vi "Config.vi"() -> ()   [LabVIEW 2020]
uses:
  Global_Variable/Global.vi
  Global_Variable/A180648.vi
  <vilib>/Utility/config.llb/NI_LVConfig.lvlib
  Libraries/S7/S7.lvlib
panel:
  in  "实验项":T1
  in  "滑移力复测":bool
  in  "产品型号":string(combo)
  in  "删除":bool
  in  "确定":bool
  in  "添加":bool
  in  "退出":bool
  in  "更新":bool
  in  "选项卡控件":enum32{"产品参数"}(tab)
  in  "结果判定参数":string[][](table)=[["mm"], ["KN"], ["KN"], ["KN"], [""], [""], [""], [""], [""], [""], [""], [""]]
  in  "判定框参数":string[][](table)=[["mm"], ["KN"], ["mm"], ["KN"]]
  in  "坐标轴参数":string[][](table)=[[""], ["°/S"], ["°"], ["Nm"]]
  # "滑移力复测及管柱总成装配台"
types:
  T1 = cluster{"第一颗螺丝":bool, "第二颗螺丝":bool, "第三颗螺丝 ":bool}
  T2 = typedef "NI_LVConfig.lvlib/Config Data RefNum.ctl" = refnum<k1>
  T3 = cluster{"[0]":cluster{string, dbl, dbl}, "[1]":cluster{string, dbl, dbl}, "[2]":cluster{string, dbl, dbl}, "[3]":cluster{string, dbl, dbl}}
  T4 = cluster{"位移":cluster{"单位":string, "下限":dbl, "上限":dbl}, "拉力":cluster{"单位":string, "下限":dbl, "上限":dbl}, "位移1":cluster{"单位":string, "下限":dbl, "上限":dbl}, "压力":cluster{"单位":string, "下限":dbl, "上限":dbl}}
  T5 = cluster{"[0]":cluster{string, dbl, dbl}, "[1]":cluster{string, dbl, dbl}, "[2]":cluster{string, dbl, dbl}, "[3]":cluster{string, dbl, dbl}, "[4]":cluster{string, dbl, dbl}, "[5]":cluster{string, dbl, dbl}}
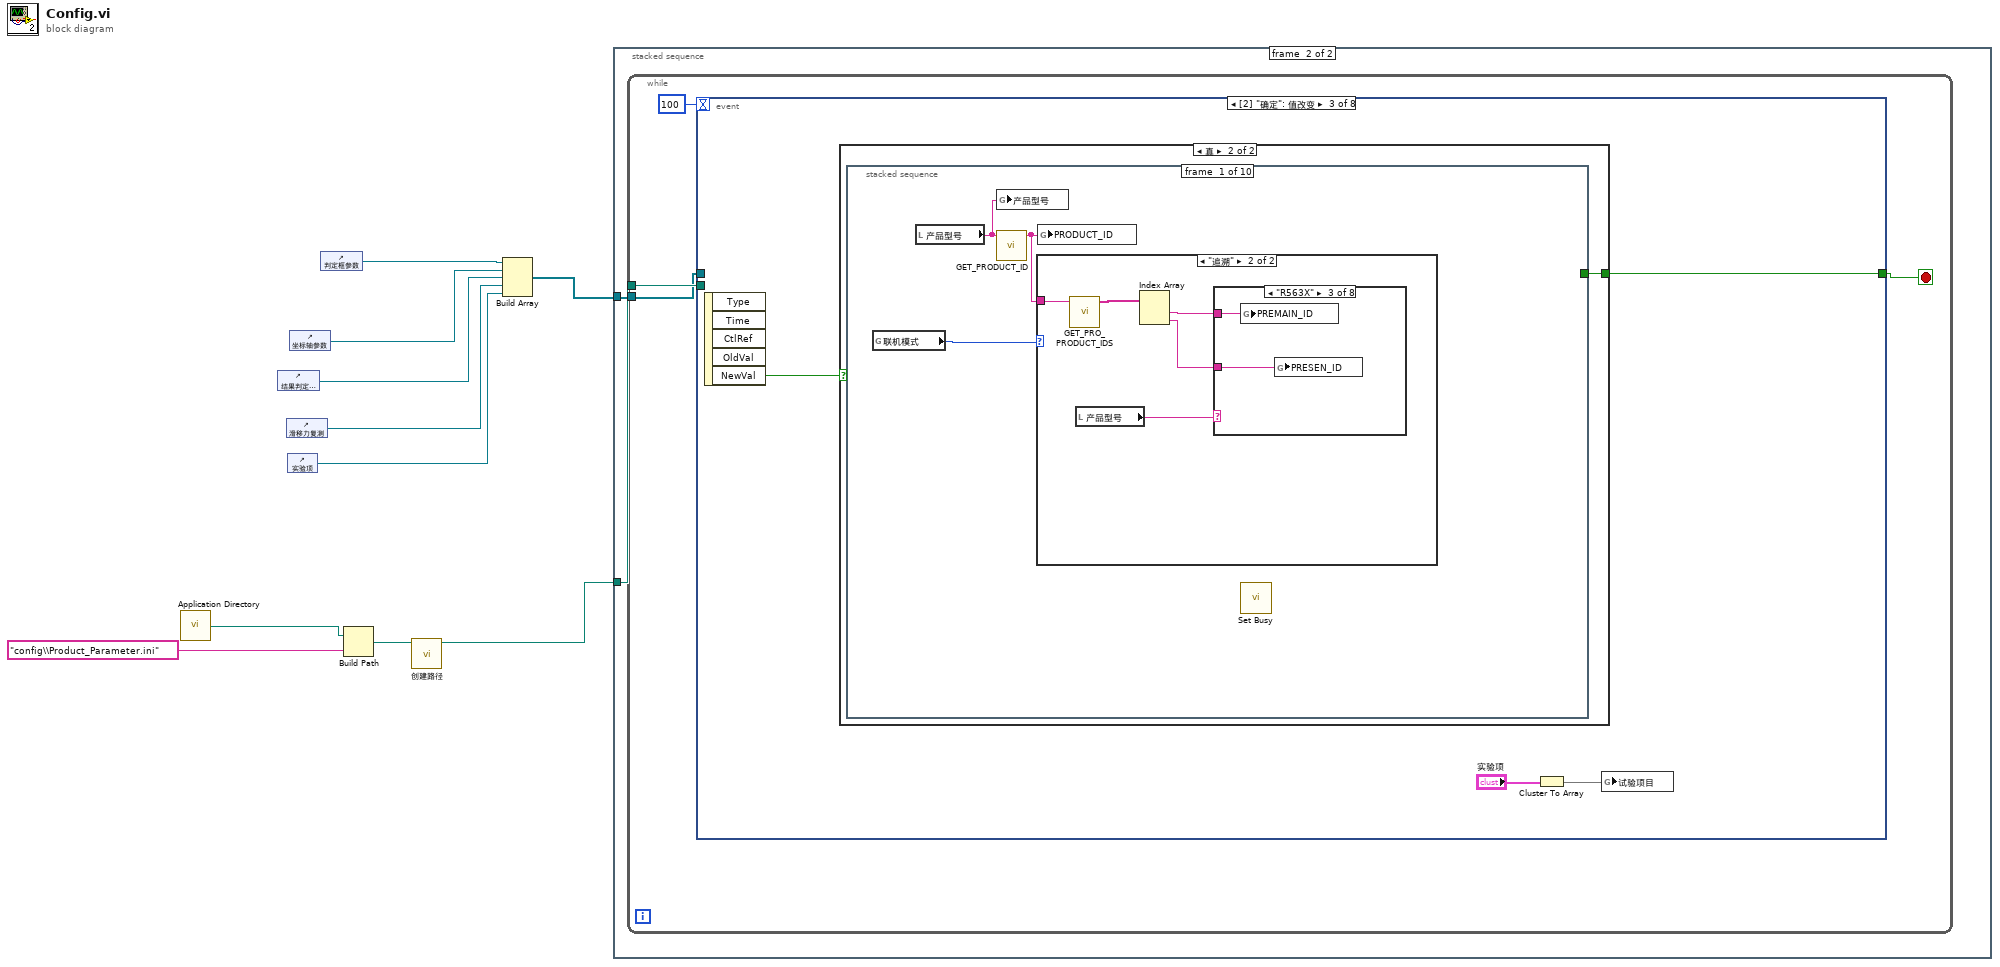
[diagram p0: block diagram]
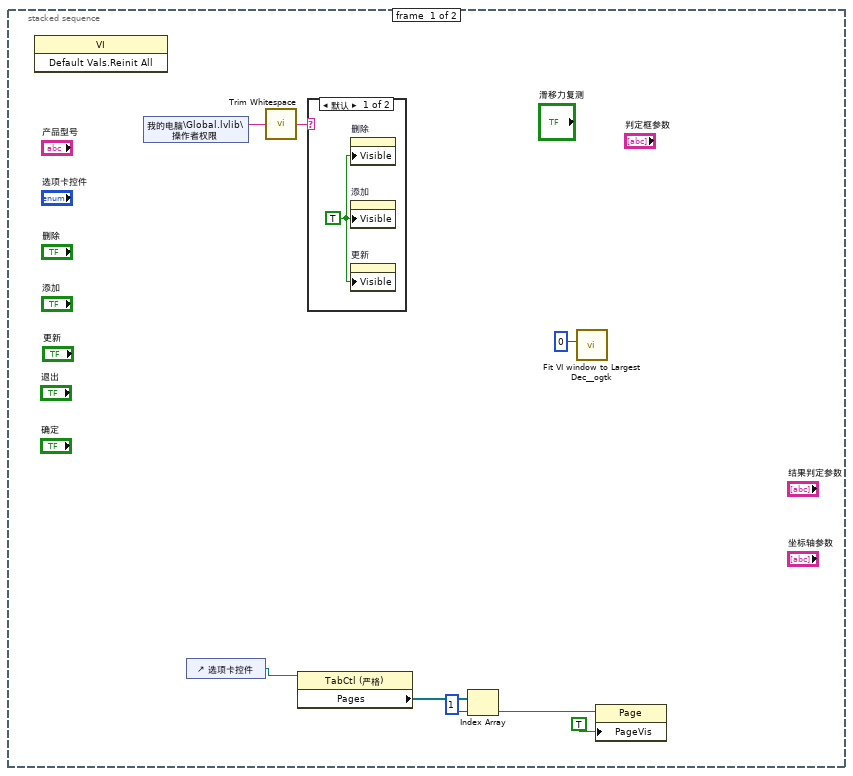
[diagram p2: hidden frame]
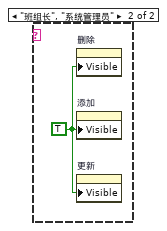
[diagram p3: hidden frame]
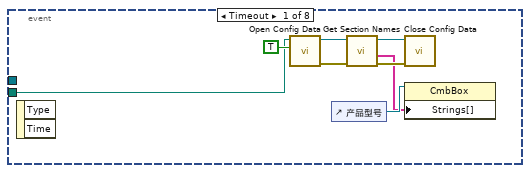
[diagram p4: hidden frame]
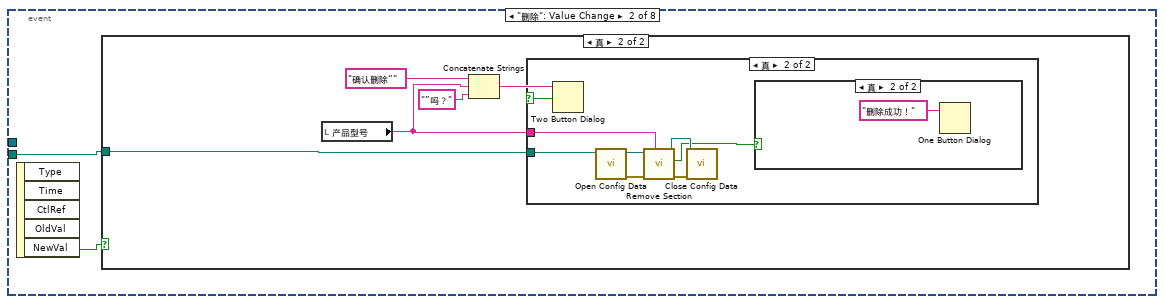
[diagram p5: hidden frame]
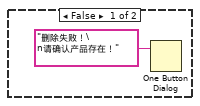
[diagram p8: hidden frame]
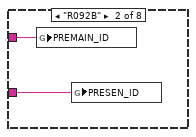
[diagram p12: hidden frame]
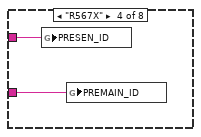
[diagram p13: hidden frame]
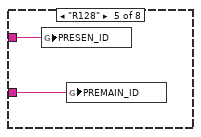
[diagram p14: hidden frame]
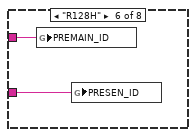
[diagram p15: hidden frame]
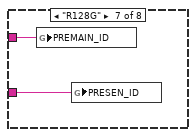
[diagram p16: hidden frame]
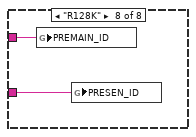
[diagram p17: hidden frame]
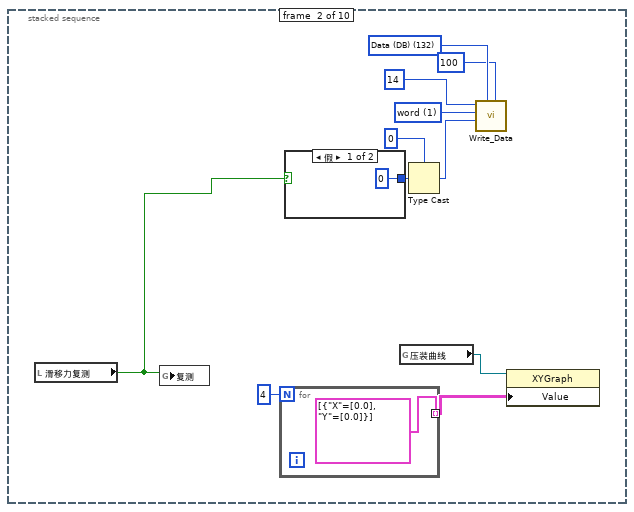
[diagram p18: hidden frame]
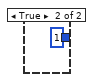
[diagram p19: hidden frame]
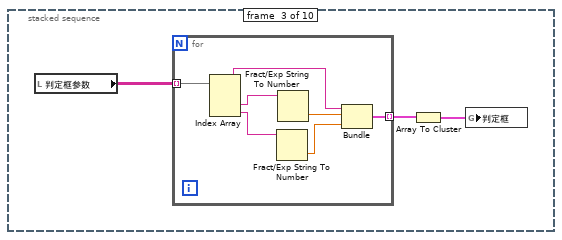
[diagram p20: hidden frame]
diagram:
  n1 = call <vilib>:"Application Directory.vi"() -> ("Application Directory"=w9:path)
  n2 = control-ref of="结果判定参数"() -> (w4:refnum<vi>)
  n3 = control-ref of="滑移力复测"() -> (w2:refnum<vi>)
  n4 = control-ref of="实验项"() -> (w1:refnum<vi>)
  n5 = control-ref of="坐标轴参数"() -> (w5:refnum<vi>)
  n6 = control-ref of="判定框参数"() -> (w3:refnum<vi>)
  n7 = Build Path(base path=w9, name or relative path="config\\Product_Parameter.ini" ("名称或相对路径")) -> (appended path=w7:path)
  n8 = call "创建路径.vi"("path"=w7) -> ("path out"=w6:path)  [unwired: 9 in, 1 out]
  n9 = Build Array(w3, w5, w4, w2, w1) -> (w10:refnum<vi>[])
  n10 = stacked-sequence {
    tunnel: w10 -> [_ w22]
    tunnel: w6 -> [_ w21]
    frame #0 {
      n11 = invoke class="VI" method="Default Vals.Reinit All"() -> ()  [unwired: 3 in, 3 out]
      n12 = shared-variable "我的电脑\\Global.lvlib\\操作者权限"() -> (w18:string)  [unwired: 1 in, 1 out]
      n13 = control-ref of="选项卡控件"() -> (w15:refnum<vi>)
      n14 = call <vilib>:"Trim Whitespace.vi"("string"=w18) -> ("trimmed string"=w17:string)  [unwired: 1 in]
      n15 = property class="TabCtl (严格)"(reference=w15) -> ("Pages"=w14:refnum<vi>[])  [unwired: 1 in, 2 out]
      n16 = case shown="默认" w17 {
        frame Default {
          w19 = TRUE ("可见")
          n17 = property on="删除" class="Bool (严格)"("Visible"=w19) -> ()  [unwired: 2 in, 2 out]
          n18 = property on="添加" class="Bool (严格)"("Visible"=w19) -> ()  [unwired: 2 in, 2 out]
          n19 = property on="更新" class="Bool (严格)"("Visible"=w19) -> ()  [unwired: 2 in, 2 out]
        }
        frame "班组长", "系统管理员" {
          w20 = TRUE ("可见")
          n20 = property on="删除" class="Bool (严格)"("Visible"=w20) -> ()  [unwired: 2 in, 2 out]
          n21 = property on="添加" class="Bool (严格)"("Visible"=w20) -> ()  [unwired: 2 in, 2 out]
          n22 = property on="更新" class="Bool (严格)"("Visible"=w20) -> ()  [unwired: 2 in, 2 out]
        }
      }
      n23 = Index Array(array=w14, index=1 ("索引")) -> (element=w13:refnum<vi>)
      n24 = call <userlib>:"Fit VI window to Largest Dec__ogtk.vi"("border spacing (2 px)"=0) -> ()  [unwired: 5 in, 2 out]
      n25 = property class="Page"(reference=w13, "PageVis"=TRUE ("选项卡可见")) -> ()  [unwired: 1 in, 2 out]
    }
    frame #1 {
      n26 = while {
        tunnel: w21 -> [w26]
        tunnel: w22 -> [w24]
        stop <- w25 stop-if-true
        n27 = event shown="[2] \"确定\": 值改变" {
          selector: _ -> [_ _ _ _ _ _ _ _]
          dyn-events: _ -> [_ _ _ _ _ _ _ _]
          timeout: 100 -> [_ _ _ _ _ _ _ _]
          tunnel: w26 -> [w29 w36 _ w158 w185 _ w209 _]
          tunnel: [_ _ w54 _ _ TRUE _ TRUE] -> w25
          tunnel: w24 -> [_ _ _ w159 w186 _ w208 _]
          event Timeout {
            n28 = event-data() -> ()  [unwired: 1 in, 2 out]
            n29 = call <vilib>:"Open Config Data.vi"("create file if necessary (T)"=TRUE, "configuration file path"=w29) -> ("error out"=w31:errorcluster, "refnum"=w30:T2)  [unwired: 7 in, 1 out]
            n30 = control-ref of="产品型号"() -> (w28:refnum<vi>)
            n31 = call <vilib>:"Get Section Names.vi"("error in (no error)"=w31, "refnum"=w30) -> ("error out"=w33:errorcluster, "section names"=w27:string[], "refnum out"=w32:T2)  [unwired: 7 in]
            n32 = call <vilib>:"Close Config Data.vi"("error in (no error)"=w33, "refnum"=w32) -> ()  [unwired: 8 in, 2 out]
            n33 = property on="属性节点" class="CmbBox"(reference=w28, "Strings[]"=w27) -> ()  [unwired: 1 in, 2 out]
          }
          event "删除": Value Change {
            n34 = event-data() -> ("NewVal"=w35:bool)  [unwired: 1 in, 4 out]
            n35 = case shown="真" w35 {
              tunnel: w36 -> [_ w38]
              frame False {
              }
              frame True {
                n36 = local read "产品型号"() -> (w37:string)
                n37 = Concatenate Strings("确认删除“", w37, "”吗？") -> (w40:string)
                n38 = Two Button Dialog(message=w40) -> (T button?=w39:bool)  [unwired: 2 in]
                n39 = case shown="真" w39 {
                  tunnel: w38 -> [_ w44]
                  tunnel: w37 -> [_ w43]
                  frame False {
                  }
                  frame True {
                    n40 = call <vilib>:"Open Config Data.vi"("configuration file path"=w44) -> ("error out"=w46:errorcluster, "refnum"=w49:T2)  [unwired: 8 in, 1 out]
                    n41 = call <vilib>:"Remove Section.vi"("section"=w43, "error in (no error)"=w46, "refnum"=w49) -> ("error out"=w48:errorcluster, "section exists?"=w45:bool, "refnum out"=w47:T2)  [unwired: 6 in]
                    n42 = call <vilib>:"Close Config Data.vi"("error in (no error)"=w48, "refnum"=w47) -> ()  [unwired: 8 in, 2 out]
                    n43 = case shown="真" w45 {
                      frame False {
                        n44 = One Button Dialog(message="删除失败！\n请确认产品存在！" ("消息")) -> ()  [unwired: 1 in, 1 out]
                      }
                      frame True {
                        n45 = One Button Dialog(message="删除成功！" ("消息")) -> ()  [unwired: 1 in, 1 out]
                      }
                    }
                  }
                }
              }
            }
          }
          event "确定": Value Change {
            n46 = event-data() -> ("NewVal"=w55:bool)  [unwired: 1 in, 4 out]
            n47 = case shown="真" w55 {
              tunnel: [_ w56] -> w54
              frame False {
              }
              frame True {
                n48 = stacked-sequence {
                  tunnel: [_ _ _ _ _ _ _ _ _ TRUE] -> w56
                  frame #0 {
                    n49 = global read "Global.vi" "联机模式"() -> (w57:enum16{"单机", "追溯"})
                    n50 = local read "产品型号"() -> (w59:string)
                    n51 = global write "Global.vi" "产品型号"(w59) -> ()
                    n52 = call "GET_PRODUCT_ID.vi"("PRODFUCT_NAME"=w59) -> ("PRODUCT_ID"=w58:string)  [unwired: 10 in]
                    n53 = case shown="\"追溯\"" w57 {
                      tunnel: w58 -> [_ w64]
                      frame "单机", Default {
                      }
                      frame "追溯" {
                        n54 = call "GET_PRO_PRODUCT_IDS.vi"("PRODUCT_ID"=w64) -> ("前序工位"=w63:string[])  [unwired: 10 in]
                        n55 = local read "产品型号"() -> (w60:string)
                        n56 = Index Array(array=w63) -> (element #1=w62:string, element #2=w61:string)  [unwired: 2 in]
                        n57 = case shown="\"R563X\"" w60 {
                          tunnel: w62 -> [_ w66 w68 w70 w72 w74 w76 w78]
                          tunnel: w61 -> [_ w65 w67 w69 w71 w73 w75 w77]
                          frame "假", Default {
                          }
                          frame "R092B" {
                            n58 = global write "追溯Global.vi" "PREMAIN_ID"(w66) -> ()
                            n59 = global write "追溯Global.vi" "PRESEN_ID"(w65) -> ()
                          }
                          frame "R563X" {
                            n60 = global write "追溯Global.vi" "PREMAIN_ID"(w68) -> ()
                            n61 = global write "追溯Global.vi" "PRESEN_ID"(w67) -> ()
                          }
                          frame "R567X" {
                            n62 = global write "追溯Global.vi" "PRESEN_ID"(w70) -> ()
                            n63 = global write "追溯Global.vi" "PREMAIN_ID"(w69) -> ()
                          }
                          frame "R128" {
                            n64 = global write "追溯Global.vi" "PRESEN_ID"(w72) -> ()
                            n65 = global write "追溯Global.vi" "PREMAIN_ID"(w71) -> ()
                          }
                          frame "R128H" {
                            n66 = global write "追溯Global.vi" "PREMAIN_ID"(w74) -> ()
                            n67 = global write "追溯Global.vi" "PRESEN_ID"(w73) -> ()
                          }
                          frame "R128G" {
                            n68 = global write "追溯Global.vi" "PREMAIN_ID"(w76) -> ()
                            n69 = global write "追溯Global.vi" "PRESEN_ID"(w75) -> ()
                          }
                          frame "R128K" {
                            n70 = global write "追溯Global.vi" "PREMAIN_ID"(w78) -> ()
                            n71 = global write "追溯Global.vi" "PRESEN_ID"(w77) -> ()
                          }
                        }
                      }
                    }
                    n72 = global write "追溯Global.vi" "PRODUCT_ID"(w58) -> ()
                    n73 = call <vilib>:"Set Busy.vi"() -> ()  [unwired: 10 in, 2 out]
                  }
                  frame #1 {
                    w84 = u16 1 items=["byte", "word", "Dword"] ("数据类型")
                    w86 = u8 132 items=["I/O (P)"=128, "Input (I)"=129, "Output (Q)"=130, "Bit Memory (M)"=131, "Data (DB)"=132, "Instance Data (DI)"=133, "Local Data (L)"=134, "Predecessor Local Data (VL)"=135] ("寄存器类型")
                    n74 = local read "滑移力复测"() -> (w79:bool)
                    n75 = global write "Global.vi" "复测"(w79) -> ()
                    n76 = for {
                      N: 4 -> [_]
                      tunnel: [cluster{"X":dbl[], "Y":dbl[]}[] [{"X"=[0.0], "Y"=[0.0]}]] -> w89 mode=indexing
                    }
                    n77 = case shown="假" w79 {
                      tunnel: [0 ("x") 1 ("x")] -> w80
                      frame False {
                      }
                      frame True {
                      }
                    }
                    n78 = global read "A180648.vi" "压装曲线"() -> (w87:refnum<vi>)
                    n79 = Type Cast(type=u32 0 ("写入地址"), x=w80) -> (*(type *) &x=w82:u32)
                    n80 = call "Write_Data.vi"("DB #"=u16 100, "寄存器类型"=w86, "写入数据"=w82, "数据类型"=w84, "写入地址"=u32 14) -> ()  [unwired: 4 in, 3 out]
                    n81 = property class="XYGraph"(reference=w87, "Value"=w89) -> ()  [unwired: 1 in, 2 out]
                  }
                  frame #2 {
                    n82 = local read "判定框参数"() -> (w95:string[][])
                    n83 = for {
                      tunnel: w95 -> [w102] mode=indexing
                      tunnel: [w96] -> w94 mode=indexing
                      n84 = Index Array(array=w102) -> (element #1=w99:string, element #2=w101:string, element #3=w100:string)  [unwired: 3 in]
                      n85 = Fract/Exp String To Number(string=w100) -> (number=w97:dbl)  [unwired: 3 in, 1 out]
                      n86 = Fract/Exp String To Number(string=w101) -> (number=w98:dbl)  [unwired: 3 in, 1 out]
                      n87 = Bundle(w99, w98, w97) -> (w96:cluster{string, dbl, dbl})  [unwired: 1 in]
                    }
                    n88 = Array To Cluster(array=w94) -> (cluster=w93:T3)
                    n89 = global write "判定参数.vi" "判定框"(w93) -> ()
                  }
                  frame #3 {
                    n90 = global read "A180648.vi" "压装曲线"() -> (w109:refnum<vi>)
                    n91 = property class="XYGraph"(reference=w109) -> (reference out=w106:refnum<vi>, "Value"=w108:variant)  [unwired: 1 in, 1 out]
                    n92 = Variant To Data(type=cluster{"X":dbl[], "Y":dbl[]}[] [{"X"=[], "Y"=[]}], Variant=w108) -> (data=w107:cluster{"X":dbl[], "Y":dbl[]}[])  [unwired: 1 in, 1 out]
                    n93 = global read "判定参数.vi" "判定框"() -> (w103:T4)
                    n94 = for {
                      tunnel: w107 -> [w112] mode=indexing
                      tunnel: [w111] -> w104 mode=indexing
                      tunnel: w103 -> [w110]
                      i -> [w113]
                      n95 = case shown="1" w113 {
                        tunnel: w112 -> [w114 _ _]
                        tunnel: [w114 w117 w127] -> w111
                        tunnel: w110 -> [_ w122 w128]
                        frame Default {
                        }
                        frame 0 {
                          n96 = Unbundle By Name(w122) -> ("位移.下限"=w121:dbl, "位移.上限"=w120:dbl, "压力.下限"=w115:dbl, "压力.上限"=w116:dbl)
                          n97 = Build Array(w120, w120, w121, w121, w120) -> (w119:dbl[])
                          n98 = Build Array(w115, w116, w116, w115, w115) -> (w118:dbl[])
                          n99 = Bundle(w119, w118) -> (w117:cluster{dbl[], dbl[]})  [unwired: 1 in]
                        }
                        frame 1 {
                          n100 = Unbundle By Name(w128) -> ("位移.下限"=w132:dbl, "位移.上限"=w131:dbl, "压力.上限"=w125:dbl, "压力.下限"=w126:dbl)
                          n101 = Negate(x=w126) -> (-x=w123:dbl)
                          n102 = Negate(x=w125) -> (-x=w124:dbl)
                          n103 = Build Array(w131, w131, w132, w132, w131) -> (w130:dbl[])
                          n104 = Build Array(w124, w123, w123, w124, w124) -> (w129:dbl[])
                          n105 = Bundle(w130, w129) -> (w127:cluster{dbl[], dbl[]})  [unwired: 1 in]
                        }
                      }
                    }
                    n106 = property class="XYGraph"(reference=w106, "Value"=w104) -> ()  [unwired: 1 in, 2 out]
                  }
                  frame #4 {
                    n107 = local read "结果判定参数"() -> (w135:string[][])
                    n108 = for {
                      tunnel: w135 -> [w137] mode=indexing
                      tunnel: [w136] -> w133 mode=indexing
                      n109 = Index Array(array=w137) -> (element #1=w142:string, element #2=w141:string, element #3=w139:string)  [unwired: 3 in]
                      n110 = Fract/Exp String To Number(string=w141) -> (number=w140:dbl)  [unwired: 3 in, 1 out]
                      n111 = Fract/Exp String To Number(string=w139) -> (number=w138:dbl)  [unwired: 3 in, 1 out]
                      n112 = Bundle(w142, w140, w138) -> (w136:cluster{string, dbl, dbl})  [unwired: 1 in]
                    }
                    n113 = Array To Cluster(array=w133) -> (cluster=w134:T5)
                    n114 = global write "判定参数.vi" "拉压判定参数"(w134) -> ()
                  }
                  frame #5 {
                    n115 = disable-structure shown="禁用" {
                      frame Disabled {
                        n116 = local read item#-1() -> (w147)
                        n117 = Index Array(array=w147, index (col)=0 ("禁用的索引 (列)")) -> (element=w145)  [unwired: 1 in]
                        n118 = Index Array(array=w145) -> (element #1=w144, element #2=w143)  [unwired: 2 in]
                        n119 = global write "Global.vi" "软件版本号"(w144) -> ()
                        n120 = global write "Global.vi" "硬件版本号"(w143) -> ()
                      }
                      frame Enabled {
                      }
                    }
                  }
                  frame #6 {
                    n121 = call <vilib>:"Unset Busy.vi"() -> ()  [unwired: 11 in, 1 out]
                  }
                  frame #7 {
                    n122 = global read "Global.vi" "更换产品"() -> (w151:refnum<vi>)
                    n123 = global read "Global.vi" "更改标尺"() -> (w148:refnum<vi>)
                    n124 = vi-ref "Auto_Step.vi"() -> (w150:refnum<vi>)
                    n125 = vi-ref "Auto.vi"() -> (w149:refnum<vi>)
                    n126 = property class="VIRef"(reference=w151, "Val(Sgnl)"=w150) -> ()  [unwired: 1 in, 2 out]
                    n127 = property class="VIRef"(reference=w148, "Val(Sgnl)"=w149) -> ()  [unwired: 1 in, 2 out]
                  }
                  frame #8 {
                    w153 = 64 items=["None"=0, "Hand, Error, Stop"=16, "Question"=32, "Exclamation, Warning"=48, "Asterisk, Information"=64] ("icon")
                    w152 = "参数装载成功！" ("消息")
                    n128 = call "浮动通知.vi"("通知内容"=w152) -> ()  [unwired: 11 in]
                    n129 = call "信息框（标题、文本、图标）.vi"("icon"=w153, "caption"="参数加载", "text"=w152) -> ()  [unwired: 7 in, 2 out]
                  }
                  frame #9 {
                    n130 = control-ref of="本VI"() -> (w155:refnum<vi>)
                    n131 = invoke class="VI" method="FP.Close"(reference=w155) -> ()  [unwired: 2 in, 3 out]
                  }
                }
              }
            }
            n132 = Cluster To Array(cluster="实验项") -> (array=w52:bool[])
            n133 = global write "Global.vi" "试验项目"(w52) -> ()
          }
          event "添加": Value Change {
            n134 = event-data() -> ("NewVal"=w157:bool)  [unwired: 1 in, 4 out]
            n135 = case shown="真" w157 {
              tunnel: w159 -> [_ w163]
              tunnel: w158 -> [_ w162]
              frame False {
              }
              frame True {
                n136 = call "产品添加提示：用户输入"() -> ("产品型号"=w160:string, "确定"=w161:bool)  [unwired: 17 in, 1 out]
                n137 = case shown="真" w161 {
                  tunnel: w163 -> [_ w166]
                  tunnel: w162 -> [_ w165]
                  tunnel: w160 -> [_ w164]
                  frame False {
                  }
                  frame True {
                    n138 = case shown="默认" w164 {
                      selector: w164 -> [_ w169]
                      tunnel: w166 -> [_ w172]
                      tunnel: w165 -> [_ w171]
                      frame "" {
                        n139 = One Button Dialog(message="产品名称不得为空!" ("text")) -> ()  [unwired: 1 in, 1 out]
                      }
                      frame Default {
                        n140 = property on="产品型号" class="CmbBox"() -> ("Strings[]"=w170:string[])  [unwired: 2 in, 2 out]
                        n141 = Search 1D Array(1D array=w170, element=w169) -> (index of element=w168:i32)  [unwired: 1 in]
                        n142 = case shown="-1" w168 {
                          tunnel: w172 -> [_ w176]
                          tunnel: w171 -> [_ w175]
                          tunnel: w169 -> [_ w174]
                          frame Default {
                            n143 = One Button Dialog(message="产品已存在！" ("消息")) -> ()  [unwired: 1 in, 1 out]
                          }
                          frame -1 {
                            n144 = stacked-sequence {
                              tunnel: w176 -> [w182 _]
                              tunnel: w175 -> [w181 _]
                              tunnel: w174 -> [w180 _]
                              frame #0 {
                                n145 = call <vilib>:"Set Busy.vi"() -> ("error out"=w178:errorcluster)  [unwired: 10 in, 1 out]
                                n146 = call "Read_Write INI File.vi"("Mode"=enum16{"Read", "Write"}."Write", "Section"=w180, "error in"=w178, "Filepath"=w181, "Ctl Refnum"=w182) -> ("error out"=w177:errorcluster)  [unwired: 6 in]
                                n147 = call <vilib>:"Unset Busy.vi"("error in (no error)"=w177) -> ()  [unwired: 10 in, 1 out]
                              }
                              frame #1 {
                                n148 = One Button Dialog(message="添加成功！" ("消息")) -> ()  [unwired: 1 in, 1 out]
                              }
                            }
                          }
                        }
                      }
                    }
                  }
                }
              }
            }
          }
          event "产品型号": Value Change {
            n149 = event-data() -> ("NewVal"=w184:string)  [unwired: 1 in, 4 out]
            n150 = stacked-sequence {
              tunnel: w186 -> [_ _ w190]
              tunnel: w185 -> [_ _ w189]
              tunnel: w184 -> [_ w188 _]
              frame #0 {
                n151 = control-ref of="本VI"() -> (w187:refnum<vi>)
                n152 = invoke class="VI" method="Default Vals.Reinit All"(reference=w187) -> ()  [unwired: 2 in, 3 out]
              }
              frame #1 {
                n153 = local write "产品型号"(w188) -> ()
              }
              frame #2 {
                n154 = disable-structure shown="启用" {
                  disable-tunnel: w190 -> [w192 w201]
                  disable-tunnel: w189 -> [w191 w202]
                  frame Disabled {
                    n155 = for {
                      tunnel: w192 -> [w195] mode=indexing
                      tunnel: w191 -> [w194]
                      n156 = local read "产品型号"() -> (w193:string)
                      n157 = call "Read_Write ParaINI File.vi"("Mode"=enum16{"Read", "Write"}."Read", "Section"=w193, "Filepath"=w194, "Ctl Refnum"=w195) -> ()  [unwired: 7 in, 1 out]
                    }
                  }
                  frame Enabled {
                    n158 = call <vilib>:"Set Busy.vi"() -> ("error out"=w197:errorcluster)  [unwired: 10 in, 1 out]
                    n159 = local read "产品型号"() -> (w200:string)
                    n160 = call "Read_Write INI File.vi"("Mode"=enum16{"Read", "Write"}."Read", "Section"=w200, "error in"=w197, "Filepath"=w202, "Ctl Refnum"=w201) -> ("error out"=w198:errorcluster)  [unwired: 6 in]
                    n161 = call <vilib>:"Unset Busy.vi"("error in (no error)"=w198) -> ()  [unwired: 10 in, 1 out]
                  }
                }
              }
            }
          }
          event "退出": Value Change {
            n162 = event-data() -> ()  [unwired: 1 in, 5 out]
            n163 = control-ref of="本VI"() -> (w205:refnum<vi>)
            n164 = invoke class="VI" method="FP.Close"(reference=w205) -> (reference out=w203:refnum<vi>, error out=w204:errorcluster)  [unwired: 2 in, 1 out]
            n165 = Close Reference(reference=w203, error in (no error)=w204) -> ()  [unwired: 1 out]
          }
          event "更新": Value Change {
            n166 = event-data() -> ("NewVal"=w207:bool)  [unwired: 1 in, 4 out]
            n167 = case shown="真" w207 {
              tunnel: w209 -> [_ w212]
              tunnel: w208 -> [_ w211]
              frame False {
              }
              frame True {
                n168 = disable-structure shown="启用" {
                  disable-tunnel: w212 -> [w215 w226]
                  disable-tunnel: w211 -> [w214 w221]
                  disable-tunnel: [w213 w223] -> w210
                  frame Disabled {
                    n169 = for {
                      tunnel: w215 -> [w218]
                      tunnel: w214 -> [w217] mode=indexing
                      tunnel: [w216] -> w213
                      n170 = local read "产品型号"() -> (w220:string)
                      n171 = call "Read_Write ParaINI File.vi"("Mode"=enum16{"Read", "Write"}."Write", "Section"=w220, "Filepath"=w218, "Ctl Refnum"=w217) -> ("error out"=w216:errorcluster)  [unwired: 7 in]
                    }
                  }
                  frame Enabled {
                    n172 = call <vilib>:"Set Busy.vi"() -> ("error out"=w222:errorcluster)  [unwired: 10 in, 1 out]
                    n173 = local read "产品型号"() -> (w225:string)
                    n174 = call "Read_Write INI File.vi"("Mode"=enum16{"Read", "Write"}."Write", "Section"=w225, "error in"=w222, "Filepath"=w226, "Ctl Refnum"=w221) -> ("error out"=w223:errorcluster)  [unwired: 6 in]
                  }
                }
                n175 = case shown="无错误" w210 {
                  frame No Error {
                    n176 = call <vilib>:"Unset Busy.vi"() -> ()  [unwired: 11 in, 1 out]
                    n177 = Wait (ms)(milliseconds to wait=u32 500 ("等待时间（毫秒）")) -> ()  [unwired: 1 out]
                    n178 = One Button Dialog(message="更新成功！" ("通知内容")) -> ()  [unwired: 1 in, 1 out]
                  }
                  frame Error {
                    n179 = Wait (ms)(milliseconds to wait=u32 500 ("等待时间（毫秒）")) -> ()  [unwired: 1 out]
                    n180 = call "浮动通知.vi"("通知内容"="更新失败！") -> ()  [unwired: 11 in]
                  }
                }
              }
            }
          }
          event Panel Close {
            n181 = event-data() -> ()  [unwired: 1 in, 3 out]
          }
        }
      }
    }
  }
